vi "FTW-DevUtil-VIMetrics.vi"(0 "VI Ref":refnum<vi>, 11 "error in":errorcluster) -> (4 "VI Ref out":refnum<vi>, 6 "VI Metrics":T1 {"FPFlags" format="0x%08x"; "BDFlags" format="0x%08x"; "Complexity" format="%.2f"; "HistoryRevision" format="rev %d"; "Callers" format="%d callers"; "CompileTime" format="Compile: %dmsec"; "FPSize" format="FP %.1p"; "CodeSize" format="BD %.1p"}, 15 "error out":errorcluster)   [LabVIEW 2015]
panel:
  # "Inputs"
  # "Outputs"
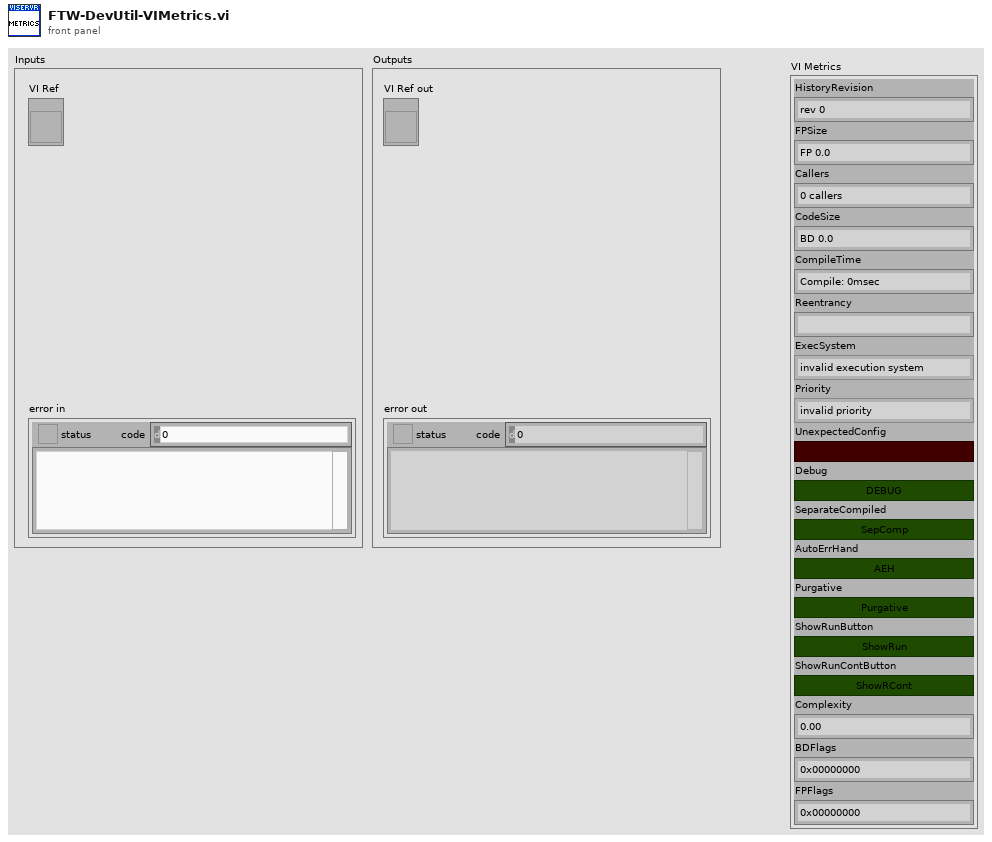
[diagram p1: front panel]
types:
  T1 = cluster{"HistoryRevision":u32, "FPSize":u32, "Callers":i32, "CodeSize":u32, "CompileTime":i32, "Reentrancy":string, "ExecSystem":enum32{"invalid execution system", "user interface", "standard", "instrument i/o", "data acquisition", "other 1", "other 2", "same as caller"}, "Priority":enum32{"invalid priority", "background priority", "normal priority", "above normal priority", "high priority", "time critical priority", "subroutine"}, "UnexpectedConfig":bool, "Debug":bool, "SeparateCompiled":bool, "AutoErrHand":bool, "Purgative":bool, "ShowRunButton":bool, "ShowRunContButton":bool, "Complexity":sgl, "BDFlags":u32, "FPFlags":u32}
  T2 = enum16{"Share clones between instances", "Preallocate clone for each instance"}
  T3 = enum32{"invalid VI type", "Standard VI", "Control VI", "Global VI", "Polymorphic VI", "Configuration VI", "SubSystem", "Facade VI", "Method VI", "Statechart Diagram VI"}
  T4 = enum32{"invalid execution system", "user interface", "standard", "instrument i/o", "data acquisition", "other 1", "other 2", "same as caller"}
  T5 = enum32{"invalid priority", "background priority", "normal priority", "above normal priority", "high priority", "time critical priority", "subroutine"}
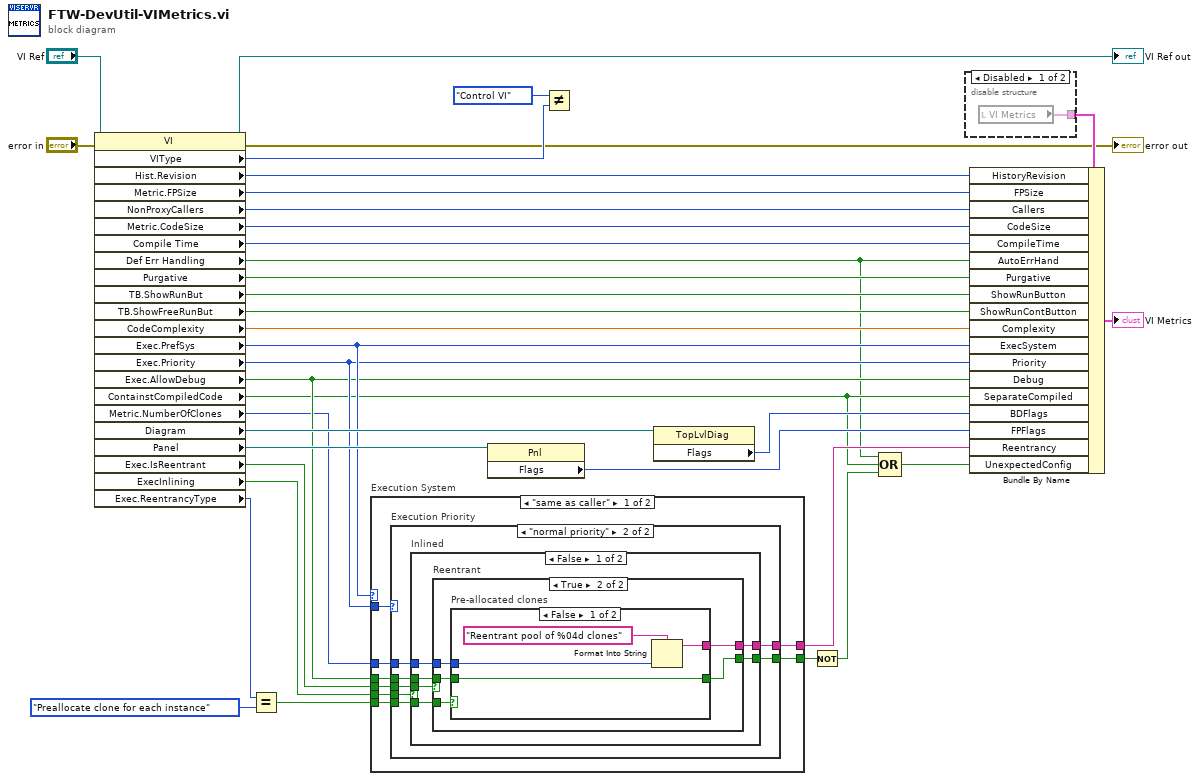
[diagram p0: block diagram]
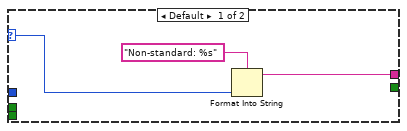
[diagram p3: hidden frame]
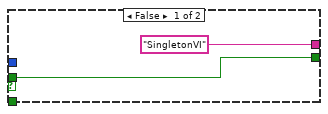
[diagram p4: hidden frame]
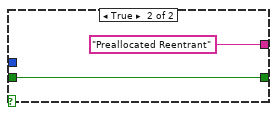
[diagram p5: hidden frame]
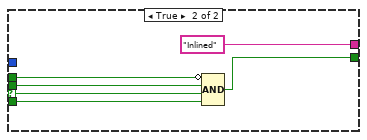
[diagram p6: hidden frame]
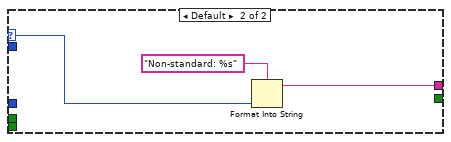
[diagram p7: hidden frame]
diagram:
  n1 = property class="VI"(reference="VI Ref", error in="error in") -> (reference out=→"VI Ref out":refnum<vi>, error out=→"error out":errorcluster, "VIType"=w35:T3, "Hist.Revision"=w15:u32, "Metric.FPSize"=w33:u32, "NonProxyCallers"=w32:i32, "Metric.CodeSize"=w24:u32, "Compile Time"=w36:i32, "Def Err Handling"=w1:bool, "Purgative"=w31:bool, "TB.ShowRunBut"=w30:bool, "TB.ShowFreeRunBut"=w29:bool, "CodeComplexity"=w5:sgl, "Exec.PrefSys"=w13:T4, "Exec.Priority"=w12:T5, "Exec.AllowDebug"=w7:bool, "ContainstCompiledCode"=w2:bool, "Metric.NumberOfClones"=w6:u32, "Diagram"=w28:refnum<vi>, "Panel"=w27:refnum<vi>, "Exec.IsReentrant"=w16:bool, "ExecInlining"=w11:bool, "Exec.ReentrancyType"=w9:T2)
  n2 = Equal?(x=w9, y=T2."Preallocate clone for each instance" ("Execution:Reentrancy Type")) -> (x = y?=w8:bool)
  n3 = case "Execution System" shown="\"same as caller\"" w13 {
    selector: w13 -> [_ w80]
    tunnel: [w43 w81] -> w23
    tunnel: [w39 _] -> w14
    tunnel: w16 -> [w40 _]
    tunnel: w11 -> [w42 _]
    tunnel: w7 -> [w41 _]
    tunnel: w8 -> [w38 _]
    tunnel: w12 -> [w44 _]
    tunnel: w6 -> [w37 _]
    frame "same as caller" {
      n4 = case "Execution Priority" shown="\"normal priority\"" w44 {
        selector: w44 -> [w46 _]
        tunnel: [w45 w50] -> w43
        tunnel: w42 -> [_ w54]
        tunnel: w41 -> [_ w53]
        tunnel: w40 -> [_ w52]
        tunnel: [_ w51] -> w39
        tunnel: w38 -> [_ w49]
        tunnel: w37 -> [_ w48]
        frame Default {
          n5 = Format Into String(format string="Non-standard: %s", w46) -> (resulting string=w45:string)  [unwired: 2 in, 1 out]
        }
        frame "normal priority" {
          n6 = case "Inlined" shown="False" w54 {
            selector: w54 -> [_ w75]
            tunnel: w53 -> [w56 w79]
            tunnel: w52 -> [w60 w78]
            tunnel: [w57 w77] -> w51
            tunnel: [w59 "Inlined"] -> w50
            tunnel: w49 -> [w58 w74]
            tunnel: w48 -> [w55 _]
            frame False {
              n7 = case "Reentrant" shown="True" w60 {
                tunnel: ["SingletonVI" w66] -> w59
                tunnel: w58 -> [_ w67]
                tunnel: [w61 w65] -> w57
                tunnel: w56 -> [w61 w64]
                tunnel: w55 -> [_ w63]
                frame False {
                }
                frame True {
                  n8 = case "Pre-allocated clones" shown="False" w67 {
                    tunnel: [w69 "Preallocated Reentrant"] -> w66
                    tunnel: [w71 w72] -> w65
                    tunnel: w64 -> [w71 w72]
                    tunnel: w63 -> [w70 _]
                    frame False {
                      n9 = Format Into String(format string="Reentrant pool of %04d clones", w70) -> (resulting string=w69:string)  [unwired: 2 in, 1 out]
                    }
                    frame True {
                    }
                  }
                }
              }
            }
            frame True {
              n10 = Compound Arithmetic op=AND(invert w79, w78, w75, w74) -> (w77:bool)
            }
          }
        }
      }
    }
    frame Default {
      n11 = Format Into String(format string="Non-standard: %s", w80) -> (resulting string=w81:string)  [unwired: 2 in, 1 out]
    }
  }
  n12 = property class="Pnl"(reference=w27) -> ("Flags"=w25:u32)  [unwired: 1 in, 2 out]
  n13 = Not Equal?(x=T3."Control VI", y=w35) -> ()  [unwired: 1 out]
  n14 = property class="TopLvlDiag"(reference=w28) -> ("Flags"=w26:u32)  [unwired: 1 in, 2 out]
  n15 = Not(x=w14) -> (.not. x?=w4:bool)
  n16 = Compound Arithmetic op=OR(w1, w2, w4) -> (w3:bool)
  n17 = disable-structure shown="Disabled" {
    disable-tunnel: [w83 _] -> w22
    frame Disabled {
      n18 = local read "VI Metrics"() -> (w83:T1)
    }
    frame Enabled {
    }
  }
  n19 = Bundle By Name(cluster=w22, "HistoryRevision"=w15, "FPSize"=w33, "Callers"=w32, "CodeSize"=w24, "CompileTime"=w36, "AutoErrHand"=w1, "Purgative"=w31, "ShowRunButton"=w30, "ShowRunContButton"=w29, "Complexity"=w5, "ExecSystem"=w13, "Priority"=w12, "Debug"=w7, "SeparateCompiled"=w2, "BDFlags"=w26, "FPFlags"=w25, "Reentrancy"=w23, "UnexpectedConfig"=w3) -> (→"VI Metrics":T1)
